vi "VD_SetVoltage.vi"(8 "error in":errorcluster, 9 "Vout2":dbl, 10 "Vout1":dbl, 11 "VISA VD_Supply":refnum<visa-resource-name>) -> (0 "error out":errorcluster, 3 "VISA VD_Supply":refnum<visa-resource-name>)   [LabVIEW 2017]
uses:
  Agilent E364X Series.lvlib
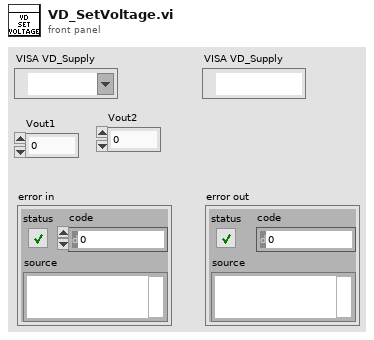
[diagram p1: front panel]
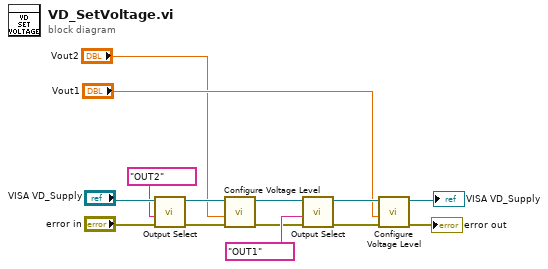
[diagram p0: block diagram]
diagram:
  n1 = call "Output Select.vi"("error in (no error)"="error in", "Instrument Select (Output 1)"="OUT2", "VISA resource name"="VISA VD_Supply") -> ("error out"=w6:errorcluster, "VISA resource name out"=w7:refnum<visa-resource-name>)  [unwired: 7 in]
  n2 = call "Configure Voltage Level.vi"("error in (no error)"=w6, "Level (0.0 Volts)"="Vout2", "VISA resource name"=w7) -> ("error out"=w5:errorcluster, "VISA resource name out"=w8:refnum<visa-resource-name>)  [unwired: 7 in]
  n3 = call "Output Select.vi"("error in (no error)"=w5, "Instrument Select (Output 1)"="OUT1", "VISA resource name"=w8) -> ("error out"=w3:errorcluster, "VISA resource name out"=w4:refnum<visa-resource-name>)  [unwired: 7 in]
  n4 = call "Configure Voltage Level.vi"("error in (no error)"=w3, "Level (0.0 Volts)"="Vout1", "VISA resource name"=w4) -> ("error out"=→"error out":errorcluster, "VISA resource name out"=→"VISA VD_Supply":refnum<visa-resource-name>)  [unwired: 7 in]
